vi "Confidence Interval (Log).vi"(0 "Y":dbl[](array[numeric]), 1 "confidence level":dbl=0.95 format="%.2f", 5 "X":dbl[](array[numeric]), 7 "Weight":dbl[](array[numeric]), 9 "amplitude":dbl, 11 "scale":dbl, 12 "base":dbl(ring)=2.71828 items=["e"=2.71828, "2"=2.0, "10"=10.0]) -> (4 "Upper Bound":dbl[](array[numeric]), 6 "Lower Bound":dbl[](array[numeric]), 8 "delta amplitude":dbl, 10 "delta scale":dbl, 15 "error":i32)   [LabVIEW 2017, in "NI_AALPro.lvlib"]
doc: "Calculates statistical intervals of the best logarithmic fit for a data set (<B>X</B>, <B>Y</B>). You must manually select the polymorphic instance to use."
uses:
  NI_AALPro.lvlib
  lvanlys.dll
panel:
  out "Coef. Lower Bound":dbl[](array[numeric])
  out "Coef. Upper Bound":dbl[](array[numeric])
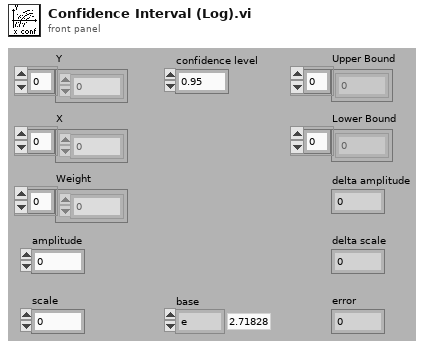
[diagram p1: front panel]
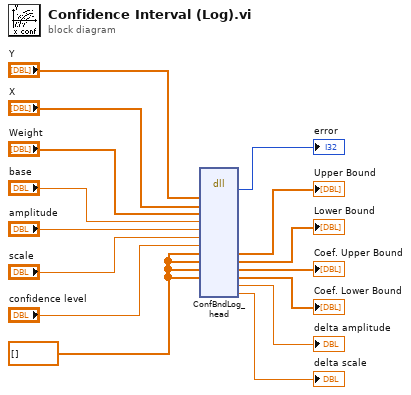
[diagram p0: block diagram]
diagram:
  w9 = dbl[] [] ("Best Linear Fit")
  n1 = dll-call lib="C:/Program Files/National Instruments/LabVIEW 2017/resource/lvanlys.*" fn="ConfBndLog_head"("y"="Y", "x"="X", "weight"="Weight", "base"="base", "amplitude"="amplitude", "scale"="scale", "confidentLevel"="confidence level", "upper"=w9, "lower"=w9, "upperCoef"=w9, "lowerCoef"=w9) -> (→"error":i32, "upper"=→"Upper Bound":dbl[], "lower"=→"Lower Bound":dbl[], "upperCoef"=→"Coef. Upper Bound":dbl[], "lowerCoef"=→"Coef. Lower Bound":dbl[], "deltaAmp"=→"delta amplitude":dbl, "deltaScl"=→"delta scale":dbl)  [unwired: 12 in, 2 out]
